vi "Twist_Angle_Net_Angle.vi"(0 "Theta_c":dbl format="%#_13g", 5 "Neck Thickness":dbl format="%#_13g", 7 "Wm":dbl format="%#_13g", 9 "Tm":dbl format="%#_13g") -> (4 "Net":dbl, 6 "Net":dbl, 8 "Sine_Net":dbl, 10 "Cosine_Net":dbl)   [LabVIEW 2019, in "Algorithm.lvclass"]
uses:
  FrameworkOverrides/Algorithm.lvclass
panel:
  out "Theta_t":dbl
  out "Theta_t":dbl
  out "W actual":dbl
  out "c":dbl
  out "b":dbl
  out "a":dbl
  out "Cos(Theta_c)":dbl
  out "Sine(Theta_c)":dbl
  out "Theta_c":dbl
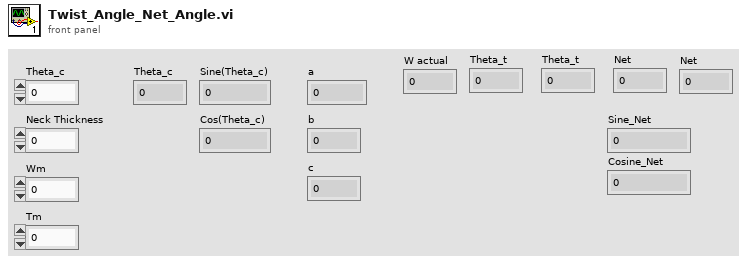
[diagram p1: front panel]
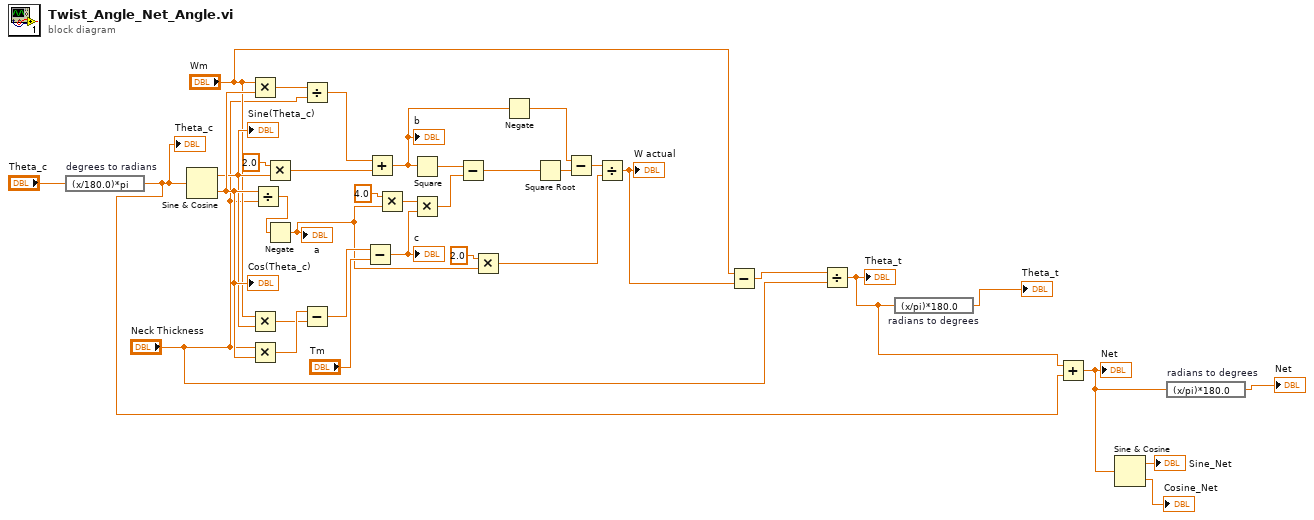
[diagram p0: block diagram]
diagram:
  n1 = expression code="(x/180.0)*pi" "degrees to radians"("Theta_c") -> (w5:dbl)
  "Theta_c" <- w5
  n2 = Sine & Cosine(0:w5) -> (1:w29:dbl, 2:w31:dbl)
  "Sine(Theta_c)" <- w29
  "Cos(Theta_c)" <- w31
  n3 = Multiply(x="Wm", y=w31) -> (x*y=w35:dbl)
  n4 = Multiply(x="Wm", y=w29) -> (x*y=w28:dbl)
  n5 = Multiply(x="Neck Thickness", y=w31) -> (x*y=w30:dbl)
  n6 = Divide(x=w31, y="Neck Thickness") -> (x/y=w13:dbl)
  n7 = Multiply(x=2.0, y=w29) -> (x*y=w32:dbl)
  n8 = Negate(x=w13) -> (-x=w12:dbl)
  "a" <- w12
  n9 = Divide(x=w35, y="Neck Thickness") -> (x/y=w34:dbl)
  n10 = Subtract(x=w30, y=w28) -> (x-y=w27:dbl)
  n11 = Subtract(x=w27, y="Tm") -> (x-y=w23:dbl)
  "c" <- w23
  n12 = Add(x=w34, y=w32) -> (x+y=w20:dbl)
  "b" <- w20
  n13 = Multiply(x=4.0, y=w12) -> (x*y=w24:dbl)
  n14 = Square(x=w20) -> (x^2=w22:dbl)
  n15 = Multiply(x=w24, y=w23) -> (x*y=w21:dbl)
  n16 = Subtract(x=w22, y=w21) -> (x-y=w14:dbl)
  n17 = Multiply(x=2.0, y=w12) -> (x*y=w15:dbl)
  n18 = Negate(x=w20) -> (-x=w19:dbl)
  n19 = Square Root(x=w14) -> (sqrt(x)=w18:dbl)
  n20 = Subtract(x=w19, y=w18) -> (x-y=w17:dbl)
  n21 = Divide(x=w17, y=w15) -> (x/y=w11:dbl)
  "W actual" <- w11
  n22 = Subtract(x="Wm", y=w11) -> (x-y=w9:dbl)
  n23 = Divide(x=w9, y="Neck Thickness") -> (x/y=w6:dbl)
  "Theta_t" <- w6
  n24 = expression code="(x/pi)*180.0" "radians to degrees"(w6) -> (→"Theta_t":dbl)
  n25 = Add(x=w6, y=w5) -> (x+y=w3:dbl)
  "Net" <- w3
  n26 = Sine & Cosine(0:w3) -> (1:→"Sine_Net":dbl, 2:→"Cosine_Net":dbl)
  n27 = expression code="(x/pi)*180.0" "radians to degrees"(w3) -> (→"Net":dbl)
